vi "Get-Set Layer Data Round Trip.vi"   [LabVIEW 2021, in "labview-icon-editor-tests.lvlib" / "layer.lvlib"]
uses:
  layer.lvlib
  source/vi.lib/LabVIEW Icon API/lv_icon/Controls/Layer.ctl
  source/vi.lib/LabVIEW Icon API/lv_icon/Classes/Layer/Layer.lvclass
  <vilib>/addons/_JKI Toolkits/Caraya/classes/Assert/Assert.lvclass
  <vilib>/addons/_JKI Toolkits/Caraya/classes/Test/Test.lvclass
types:
  T1 = typedef "Layer.ctl" = cluster{"LayerIcon":picture, "LayerName":string, "Opacity":u8, "Visibility?":bool}
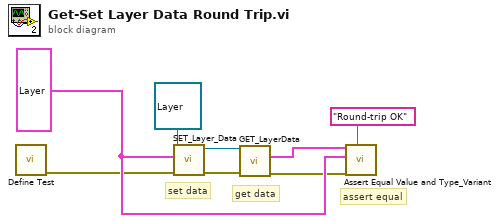
[diagram p0: block diagram]
diagram:
  w5 = T1 {"LayerIcon"=bytes[3102], "LayerName"="foo", "Opacity"=2, "Visibility?"=FALSE} ("Data")
  # "assert equal"
  # "get data"
  # "set data"
  n1 = call <vilib>:"Define Test.vi"() -> ("error out"=w1:errorcluster)  [unwired: 10 in, 1 out]
  n2 = call-dynamic "SET_Layer_Data.vi"("error in (no error)"=w1, "Data"=w5, "Layer.lvclass in"=refnum<class "Layer.lvclass"> refnum) -> ("error out"=w4:errorcluster, "Layer.lvclass out"=w8:refnum<class "Layer.lvclass">)  [unwired: 7 in]
  n3 = call-dynamic "GET_LayerData.vi"("error in (no error)"=w4, "Layer.lvclass in"=w8) -> ("error out"=w3:errorcluster, "Data"=w6:T1)  [unwired: 5 in, 3 out]
  n4 = call <vilib>:"Assert Equal Value and Type_Variant.vi"("Label"="Round-trip OK", "error in (no error)"=w3, "Y"=w5, "X"=w6) -> ()  [unwired: 6 in, 2 out]
